vi "Autonomous Independent.vi"   [LabVIEW 2018]
doc: "This VI is called when autonomous begins, and will automatically be terminated when autonomous ends. You can carry out timed or sensor driven robot movement independently without needing to return to the caller."
uses:
  <vilib>/Rock Robotics/Network Tables/NT Read String Array.vi
  Swerve/SwerveGlobals.vi
  <vilib>/Rock Robotics/Network Tables/NT Write String.vi
panel:
  # "Be sure to right-click and choose Data Operations>>Make Current Value default if you want to save the array values with the VI"
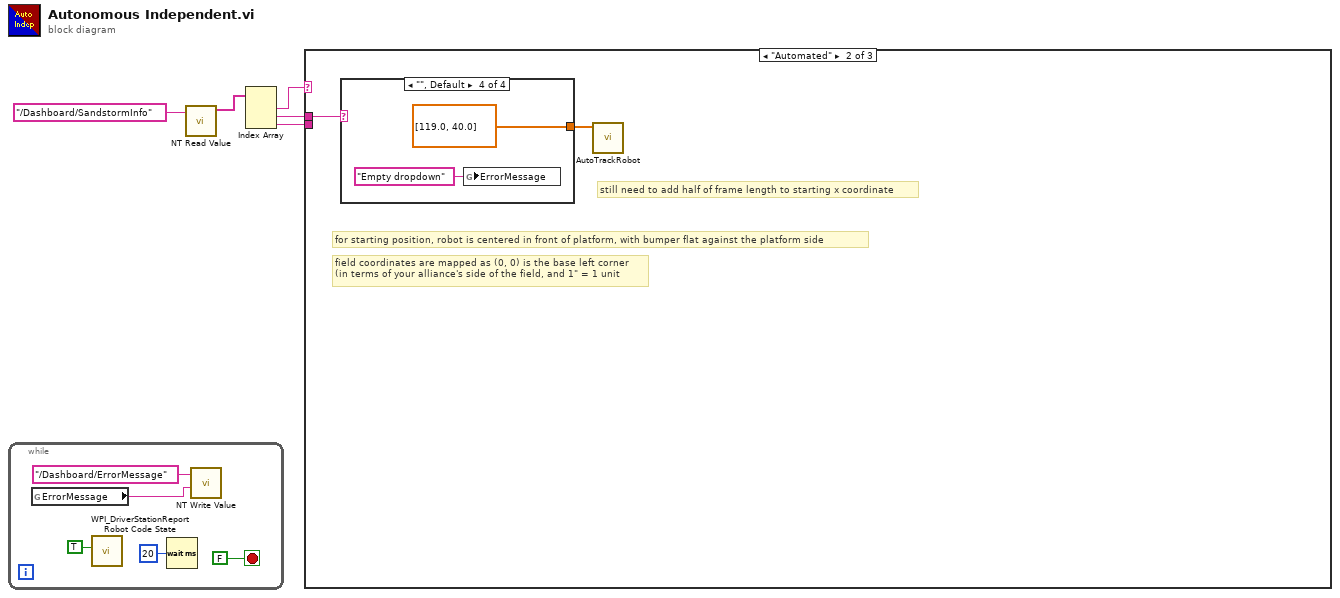
[diagram p0: block diagram]
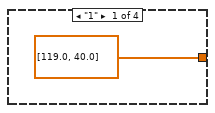
[diagram p3: hidden frame]
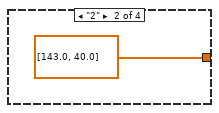
[diagram p4: hidden frame]
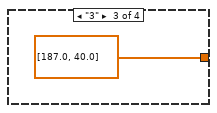
[diagram p5: hidden frame]
diagram:
  n1 = while {
    stop <- FALSE stop-if-true
    n2 = global read "SwerveGlobals.vi" "ErrorMessage"() -> (w7:string)
    n3 = call <vilib>:"WPI_DriverStationReport Robot Code State.vi"("Autonomous"=TRUE) -> ()  [unwired: 10 in, 1 out]
    n4 = Wait (ms)(milliseconds to wait=u32 20) -> ()  [unwired: 1 out]
    n5 = call-poly <vilib>:"NT Write Value.vi"("String"=w7, "Name"="/Dashboard/ErrorMessage") -> ()  [unwired: 9 in, 1 out]
  }
  n6 = call-poly <vilib>:"NT Read Value.vi"("Name"="/Dashboard/SandstormInfo") -> ("String Array"=w4:string[])  [unwired: 9 in, 1 out]
  n7 = Index Array(array=w4) -> (element #1=w3:string, element #2=w2:string, element #3=w1:string)  [unwired: 3 in]
  n8 = case shown="\"Automated\"" w3 {
    tunnel: w2 -> [_ w12 _]
    tunnel: w1 -> [_ _ _]
    frame "Manual", Default {
      # "Just the normal teleop stuff in periodic tasks"
    }
    frame "Automated" {
      # "still need to add half of frame length to starting x coordinate"
      # "for starting position, robot is centered in front of platform, with bumper flat against the platform side"
      # "field coordinates are mapped as (0, 0) is the base left corner\n(in terms of your alliance's side of the field, and 1\" = 1 unit"
      n9 = case shown="\"\", Default" w12 {
        tunnel: [dbl[] [119.0, 40.0] dbl[] [143.0, 40.0] dbl[] [187.0, 40.0] dbl[] [119.0, 40.0]] -> w11
        frame "1" {
        }
        frame "2" {
        }
        frame "3" {
        }
        frame "", Default {
          n10 = global write "SwerveGlobals.vi" "ErrorMessage"("Empty dropdown" ("ErrorMessage")) -> ()
        }
      }
      n11 = call "AutoTrackRobot.vi"("StartCoordinates"=w11) -> ()  [unwired: 10 in, 1 out]
    }
    frame "Semi-automated " {
    }
  }
